vi "Read Holding Registers.vi"(8 "error in (no error)":errorcluster, 9 "quantity":u16, 10 "starting address":u16, 11 "MB session in":refnum<class "MB_Master.lvclass">) -> (0 "error out":errorcluster, 2 "Registers":u16[](array[numeric]), 3 "MB session out":refnum<class "MB_Master.lvclass">)   [LabVIEW 2016, in "MB Master.lvlib"]
doc: "Function Code 3: Read <b>quantity</b> number of holding registers starting from <b>starting address</b>"
uses:
  MB Master.lvlib
  MB_Master.lvclass
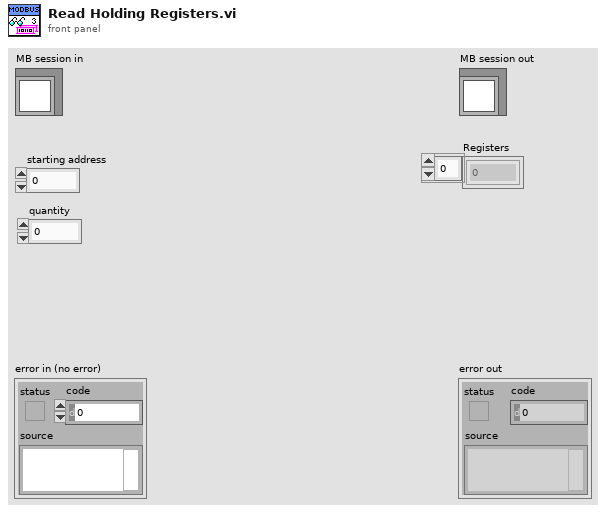
[diagram p1: front panel]
types:
  T1 = typedef "MB Master.lvlib/MB_PDU_Cluster.ctl" = cluster{"Function Code":u8, "Data":u8[], "RTU_DataBytes":i32}
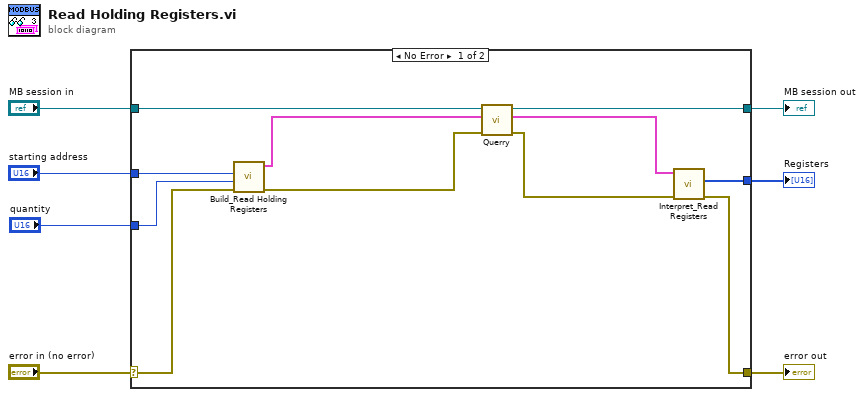
[diagram p0: block diagram]
diagram:
  n1 = case shown="No Error" "error in (no error)" {
    selector: "error in (no error)" -> [w14 w20]
    tunnel: [w13 w20] -> w6
    tunnel: [w11 w19] -> w4
    tunnel: "MB session in" -> [w10 w19]
    tunnel: "starting address" -> [w18 _]
    tunnel: "quantity" -> [w17 _]
    tunnel: [w12 _] -> w1
    frame No Error {
      n2 = call "Build_Read Holding Registers.vi"("error in (no error)"=w14, "quantity"=w17, "starting address"=w18) -> ("error out"=w15:errorcluster, "MB_PDU"=w9:T1)  [unwired: 7 in]
      n3 = call-dynamic "Querry.vi"("error in (no error)"=w15, "PDU_req"=w9, "MB_Master in"=w10) -> ("error out"=w16:errorcluster, "PDU_resp"=w8:T1, "MB_Master out"=w11:refnum<class "MB_Master.lvclass">)  [unwired: 6 in]
      n4 = call "Interpret_Read Registers.vi"("error in (no error)"=w16, "MB_PDU_resp in"=w8) -> ("error out"=w13:errorcluster, "Registers"=w12:u16[])  [unwired: 8 in]
    }
    frame Error {
    }
  }
  "error out" <- w6
  "MB session out" <- w4
  "Registers" <- w1
